vi "Auton Lift Dictation.vi"(1 "Level":dbl) -> (0 "Lift Sequence Done":bool)   [LabVIEW 2014]
uses:
  Begin/Global Variables.vi
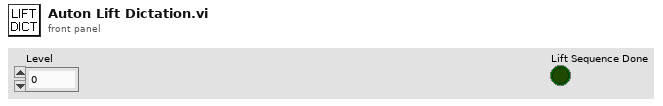
[diagram p1: front panel]
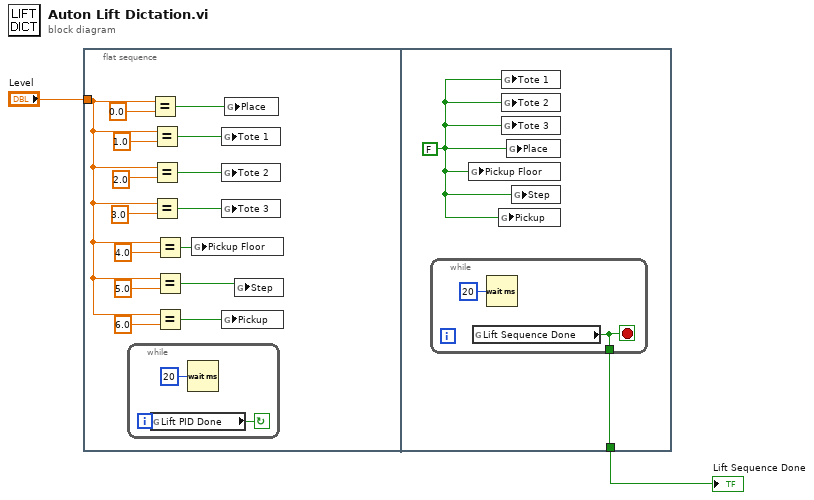
[diagram p0: block diagram]
diagram:
  n1 = flat-sequence {
    tunnel: "Level" -> [w4]
    tunnel: [w20] -> w1
    frame #0 {
      n2 = while {
        stop <- w18 continue-if-true
        n3 = global read "Global Variables.vi" "Lift PID Done"() -> (w18:bool)
        n4 = Wait (ms)(milliseconds to wait=u32 20) -> ()  [unwired: 1 out]
      }
      n5 = Equal?(x=w4, y=0.0) -> (x = y?=w14:bool)
      n6 = Equal?(x=w4, y=1.0 ("x")) -> (x = y?=w16:bool)
      n7 = Equal?(x=w4, y=2.0 ("x")) -> (x = y?=w15:bool)
      n8 = Equal?(x=w4, y=3.0 ("x")) -> (x = y?=w17:bool)
      n9 = Equal?(x=w4, y=4.0) -> (x = y?=w13:bool)
      n10 = Equal?(x=w4, y=5.0) -> (x = y?=w9:bool)
      n11 = Equal?(x=w4, y=6.0) -> (x = y?=w8:bool)
      n12 = global write "Global Variables.vi" "Pickup Floor"(w13) -> ()
      n13 = global write "Global Variables.vi" "Tote 1"(w16) -> ()
      n14 = global write "Global Variables.vi" "Tote 2"(w15) -> ()
      n15 = global write "Global Variables.vi" "Tote 3"(w17) -> ()
      n16 = global write "Global Variables.vi" "Pickup"(w8) -> ()
      n17 = global write "Global Variables.vi" "Place"(w14) -> ()
      n18 = global write "Global Variables.vi" "Step"(w9) -> ()
    }
    frame #1 {
      w21 = FALSE ("Tote 0")
      n19 = while {
        tunnel: [w22] -> w20
        stop <- w22 stop-if-true
        n20 = global read "Global Variables.vi" "Lift Sequence Done"() -> (w22:bool)
        n21 = Wait (ms)(milliseconds to wait=u32 20) -> ()  [unwired: 1 out]
      }
      n22 = global write "Global Variables.vi" "Pickup Floor"(w21) -> ()
      n23 = global write "Global Variables.vi" "Pickup"(w21) -> ()
      n24 = global write "Global Variables.vi" "Tote 1"(w21) -> ()
      n25 = global write "Global Variables.vi" "Tote 2"(w21) -> ()
      n26 = global write "Global Variables.vi" "Tote 3"(w21) -> ()
      n27 = global write "Global Variables.vi" "Place"(w21) -> ()
      n28 = global write "Global Variables.vi" "Step"(w21) -> ()
    }
  }
  "Lift Sequence Done" <- w1
